vi "Channels Configuration - Get Scan List String1.vi"(8 "error in (no error)":errorcluster, 10 "ab0":bool, 11 "Channel Array Out":string[](array[string])) -> (0 "error out":errorcluster, 3 "String":string)   [LabVIEW 2015]
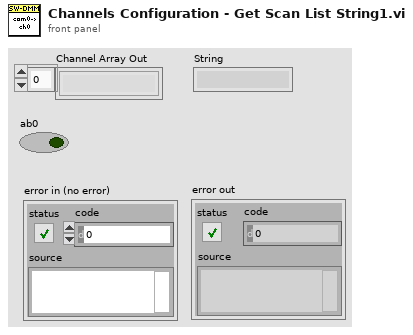
[diagram p1: front panel]
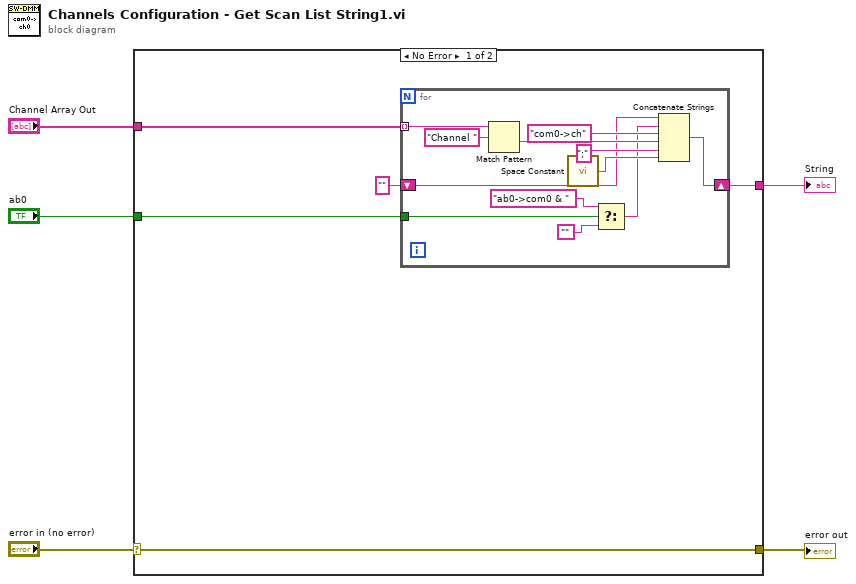
[diagram p0: block diagram]
diagram:
  n1 = case shown="No Error" "error in (no error)" {
    selector: "error in (no error)" -> [w6 w23]
    tunnel: [w10 _] -> w5
    tunnel: "ab0" -> [w9 _]
    tunnel: "Channel Array Out" -> [w7 _]
    tunnel: [w6 w23] -> w1
    frame No Error {
      n2 = for {
        tunnel: w7 -> [w22] mode=indexing
        shift-right: [w16] -> w10
        shift-left: "" -> [w13]
        tunnel: w9 -> [w15]
        n3 = Match Pattern(string=w22, regular expression="Channel ") -> (after substring=w20:string)  [unwired: 1 in, 3 out]
        n4 = call <vilib>:"Space Constant.vi"() -> ("String"=w17:string)
        n5 = Select(t="ab0->com0 & " ("Value"), s=w15, f="") -> (s? t:f=w12:string)
        n6 = Concatenate Strings(w13, w12, "com0->ch" ("string"), w20, ";" ("string"), w17) -> (w16:string)
      }
    }
    frame Error {
    }
  }
  "String" <- w5
  "error out" <- w1
